vi "HB_ThreadPool.MainDFSMTask.vi"() -> ()   [LabVIEW 2009, in "HGF_DIM_DFSM_Examples.lvlib"]
doc: "Simple application to test the HGF_ThreadPool with a simple class."
uses:
  HGF_DIM_DFSM_Examples.lvlib
  lib.lib/HGF_LVC/HGF_StateCharts/HGF_DeviceFSM/HGF_DeviceFSM_Internals.ctl
  lib.lib/HGF_LVC/HGF_StateCharts/HGF_DeviceFSM/HGF_DeviceFSM.lvsc/StatechartState.ctl
  lib.lib/HGF_LVC/HGF_StateCharts/HGF_DeviceFSM/HGF_DeviceFSM.lvsc/State.ctl
  NInstrSim/Factory/HB_DeviceFactory.lvclass
  lib.lib/HGF_LVC/HGF_BaseClasses/HGF_Factory/HGF_Factory.lvclass
  lib.lib/HGF_LVC/HGF_BaseClasses/HGF_Event/HGF_Event.lvclass
  lib.lib/HGF_LVC/HGF_BaseClasses/HGF_ThreadTask/HGF_ThreadTask.lvclass
  lib.lib/HGF_LVC/HGF_BaseClasses/HGF_NetworkVisitor/HGF_NetworkVisitor.lvclass
  lib.lib/HGF_LVC/HGF_BaseClasses/HGF_PVSubscriber/HGF_PVSubscriber.lvclass
  lib.lib/HGF_LVC/HGF_DeviceBaseClasses/HGF_DeviceVisitor/HGF_DeviceVisitor.lvclass
  lib.lib/HGF_LVC/HGF_DIM/HGF_DIMDataConverter/HGF_DIMDataConverter.lvclass
  lib.lib/HGF_LVC/HGF_DIM/HGF_DIMService/HGF_DIMService.lvclass
  lib.lib/HGF_LVC/HGF_DIM/HGF_DIMFactory/HGF_DIMFactory.lvclass/HGF_DIMFactory.lvclass
  NInstrSim/Visitors/NInstrSim_Visitor.lvclass
  lib.lib/HGF_LVC/HGF_BaseClasses/HGF_TriggeredEvent/HGF_TriggeredEvent.lvclass
  lib.lib/HGF_LVC/HGF_BaseClasses/HGF_VariantDataObject/HGF_VariantDataObject.lvclass
  lib.lib/HGF_LVC/HGF_StateCharts/HGF_DeviceFSM/HGF_DeviceFSM.lvsc/Trigger.ctl
  lib.lib/HGF_LVC/HGF_StateCharts/HGF_DFSMFactory/HGF_DFSMFactory.lvclass
  NInstrSim/Visitors/NInstrSim_ReadStatus/NInstrSim_ReadStatus.lvclass
  lib.lib/HGF_LVC/HGF_BaseClasses/HGF_Exception/HGF_Exception.lvclass
  lib.lib/HGF_LVC/HGF_BaseClasses/HGF_ThreadPool/HGF_ThreadPool.lvclass
  lib.lib/HGF_LVC/HGF_BaseClasses/HGF_Reference/HGF_Reference.lvclass
  lib.lib/HGF_LVC/HGF_Auxiliary/HGF_Auxiliary.lvlib
  lib.lib/HGF_LVC/HGF_BaseClasses/HGF_NetworkEvent/HGF_NetworkEvent.lvclass/HGF_NetworkEvent.lvclass
  lib.lib/HGF_LVC/HGF_DIM/HGF_DIMCommand/HGF_DIMCommand.lvclass
  lib.lib/DimLVEvent/LVDimInterface/LVDimInterface.lvlib
  lib.lib/HGF_LVC/HGF_DeviceBaseClasses/HGF_VISADevice/HGF_VISADevice.lvclass
  lib.lib/HGF_LVC/HGF_DeviceBaseClasses/HGF_DeviceBase/HGF_DeviceBase.lvclass
  NInstrSim/NInstrSim.lvclass
  NInstrSim/Visitors/NInstrSim_ConfigureWaveformType/NInstrSim_ConfigureWaveformType.lvclass
  lib.lib/HGF_LVC/HGF_BaseClasses/HGF_PVBase/HGF_PVBase.lvclass
  lib.lib/HGF_LVC/HGF_DIM/HGF_DIMSubscriber/HGF_DIMSubscriber.lvclass
  lib.lib/HGF_LVC/HGF_BaseClasses/HGF_Visitor/HGF_Visitor.lvclass
  lib.lib/HGF_LVC/HGF_StateCharts/HGF_DeviceFSM/HGF_DeviceFSM.lvsc
  lib.lib/HGF_LVC/HGF_StateCharts/HGF_TaskDFSM/HGF_TaskDFSM.lvclass
  lib.lib/HGF_LVC/HGF_StateCharts/HGF_DFSMVisitor/HGF_DFSMVisitor.lvclass
  lib.lib/HGF_LVC/HGF_DeviceBaseClasses/HGF_DeviceBaseClasses.lvlib
panel:
  out "Active States":T1
  out "internals":T3
  out "error code":i32
  out "no link":bool
  in  "getStatus":bool
  in  "Trigger":T4
  in  "autoConfigure":bool=TRUE
  out "exception":errorcluster
  in  "function (0:Sine)":u16(ring) items=["Sine", "Square", "Sine+Noise", "Random", "Chirp"]
  in  "Serial Configuration":T5={"Baud Rate"=9600, "Flow Control"=0, "Parity"=0, "Data Bits"=7, "Stop Bits"=10} {"Stop Bits" items=["1.0"=10, "1.5"=15, "2.0"=20]; "Data Bits" items=["7"=7, "8"=8]; "Parity" items=["None", "Odd", "Even", "Mark", "Space"]; "Flow Control" items=["None"=0, "XON/XOFF"=1, "RTS/CTS"=2, "DTR/DSR"=4]; "Baud Rate" items=["300"=300, "600"=600, "1200"=1200, "2400"=2400, "4800"=4800, "9600"=9600, "19200"=19200]}
  in  "VISA Resource Name":refnum<visa-resource-name>="GPIB0::13::INSTR"
  in  "objectName":string="myInstrSim"
  out "dcMeasurement":dbl format="%_6g"
  out "Waveform Graph":waveform(dbl)(graph)
  in  "timeout in ms (-1)":i32=3000
  out "nofTasksInQueueOut":i32
  out "nofTasksWaiting":i32
  out "autoIncrementLimit":i32=-1
  out "nofThreads":i32
  out "Default Destination timed out?":bool
  out "got object?":bool
  out "error":errorcluster
  in  "stop":bool
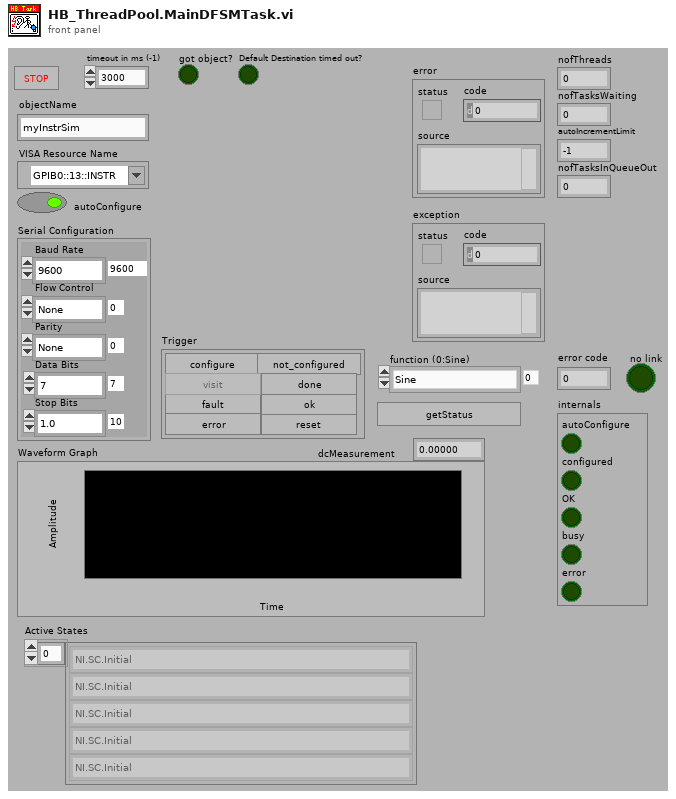
[diagram p1: front panel]
types:
  T1 = typedef "HGF_DeviceFSM.lvlib/HGF_DeviceFSM.lvsc/StatechartState.ctl" = T2[]
  T2 = typedef "HGF_DeviceFSM.lvlib/HGF_DeviceFSM.lvsc/State.ctl" = enum16{"NI.SC.Initial", "NI.SC.History", "NI.SC.ShallowHistory", "NI.SC.Terminal", "Alive", "Alive\\LiveCycle\\Configure", "Alive\\LiveCycle\\Configured", "Alive\\LiveCycle\\Error", "Alive\\LiveCycle\\NotConfigured", "Alive\\LiveCycle\\Configured\\ConfiguredRegion\\Busy", "Alive\\LiveCycle\\Configured\\ConfiguredRegion\\Idle", "Alive\\LiveCycle\\Configured\\ConfiguredRegion\\Idle\\IdleRegion\\Fault", "Alive\\LiveCycle\\Configured\\ConfiguredRegion\\Idle\\IdleRegion\\OK"}
  T3 = typedef "HGF_DeviceBaseClasses.lvlib/HGF_DeviceFSM_Internals.ctl" = cluster{"autoConfigure":bool, "configured":bool, "OK":bool, "busy":bool, "error":bool}
  T4 = cluster{"configure":bool, "visit":bool, "ok":bool, "resetError":bool, "not_configured":bool, "done":bool, "fault":bool, "error":bool}
  T5 = cluster{"Baud Rate":u32, "Flow Control":u16, "Parity":u16, "Data Bits":u16, "Stop Bits":u16}
  T6 = typedef "HGF_DeviceFSM.lvlib/HGF_DeviceFSM.lvsc/Trigger.ctl" = enum16{"NULL", "configure", "fault", "error", "resetError", "STOP", "visit", "not_configured", "done", "ok", "previsit", "configured"}
  T7 = cluster{"Boolean array[0]":bool, "Boolean array[1]":bool, "Boolean array[2]":bool, "Boolean array[3]":bool, "Boolean array[4]":bool}
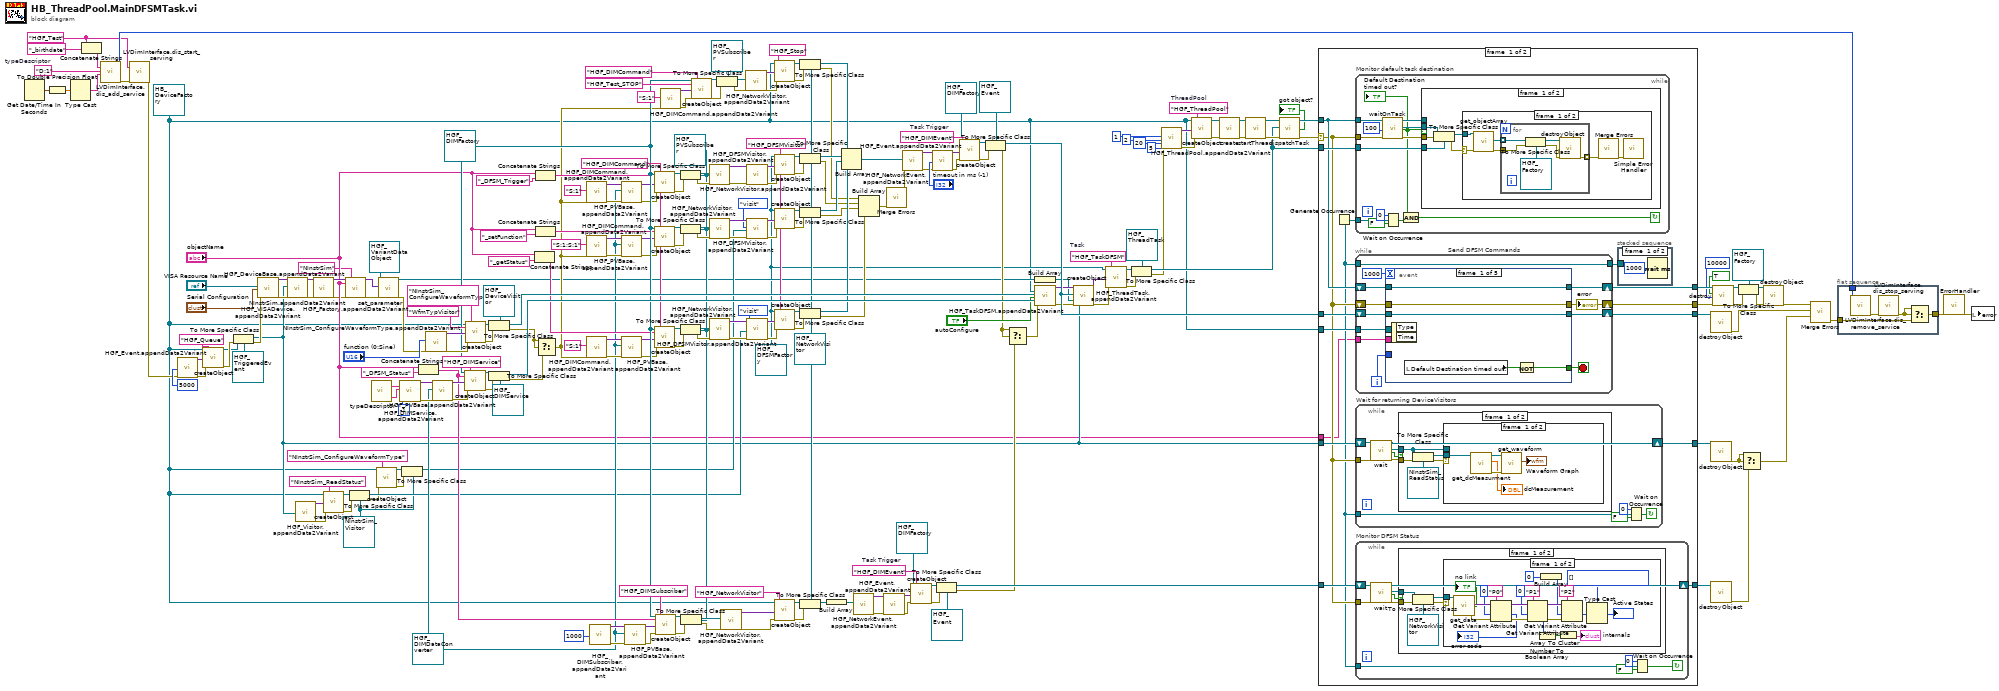
[diagram p0: block diagram]
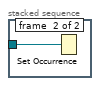
[diagram p4: hidden frame]
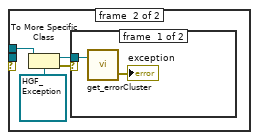
[diagram p5: hidden frame]
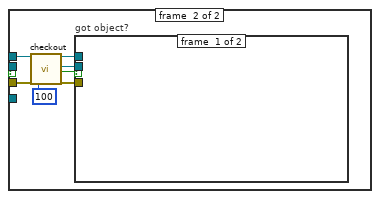
[diagram p9: hidden frame]
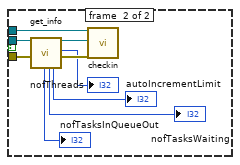
[diagram p10: hidden frame]
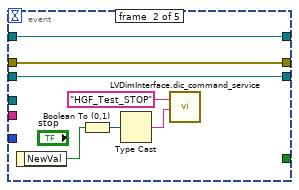
[diagram p11: hidden frame]
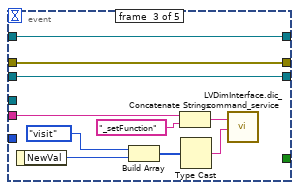
[diagram p12: hidden frame]
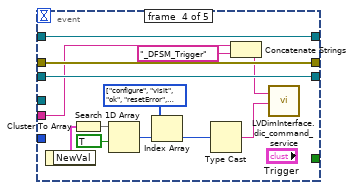
[diagram p13: hidden frame]
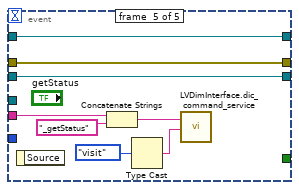
[diagram p14: hidden frame]
diagram:
  w2 = refnum<class "HGF_DFSMFactory.lvclass"> refnum ("HGF_DeviceFSM.lvlib:HGF_DFSMFactory.lvclass")
  w26 = refnum<class "NInstrSim_Visitor.lvclass"> refnum ("HB_HGF_Test.lvlib:NInstrSim_Visitor.lvclass")
  w72 = "HGF_DIMEvent"  # Task Trigger
  w58 = refnum<class "HGF_DIMFactory.lvclass"> refnum ("HGF_DIM.lvlib:HGF_DIMFactory.lvclass")
  w60 = refnum<class "HGF_PVSubscriber.lvclass"> refnum ("HGF_PVSubscriber")
  w103 = "HGF_DIMCommand" ("className")
  w90 = "HGF_DFSMVisitor" ("className")
  w35 = refnum<class "HGF_DIMDataConverter.lvclass"> refnum ("HGF_DIM.lvlib:HGF_DIMBaseType.lvclass")
  w177 = "HGF_Test" ("serverName")
  w182 = "D:1"  # typeDescriptor
  w77 = refnum<class "HGF_NetworkVisitor.lvclass"> refnum ("HGF_BaseClasses.lvlib:HGF_NetworkData.lvclass")
  w230 = "HGF_DIMEvent"  # Task Trigger
  w229 = "HGF_TaskDFSM"  # Task
  w222 = "HGF_ThreadPool"  # ThreadPool
  w1 = refnum<class "HB_DeviceFactory.lvclass"> refnum ("HB_Factory.lvclass")
  n1 = Get Date/Time In Seconds() -> (seconds since 1Jan1904=w180:timestamp)
  n2 = To Double Precision Float(number=w180) -> (double precision float=w181:dbl)
  n3 = Type Cast(x=w181) -> (*(type *) &x=w183:string)  [unwired: 1 out]
  n4 = Concatenate Strings(w177, "_birthdate") -> (w176:string)
  n5 = call "LVDimInterface.dis_add_service.vi"("serviceName"=w176, "typeDescriptor"=w182, "data"=w183) -> ("my_serviceID"=w179:i32, "error out"=w184:errorcluster)  [unwired: 2 in, 13 out]
  n6 = call "LVDimInterface.dis_start_serving.vi"("serverName"=w177, "error in (no error)"=w184) -> ("error out"=w154:errorcluster)  [unwired: 17 out]
  n7 = call "HGF_Event.appendData2Variant.vi"("timeout in ms (-1)"=5000, "error in (no error)"=w154) -> ("dup initData"=w165:variant, "error out"=w166:errorcluster)  [unwired: 1 in, 15 out]
  n8 = call "createObject.vi"("HGF_Factory"=w1, "initializationData"=w165, "error in (no error)"=w166, "className"="HGF_Queue") -> ("HGF_Object"=w162:refnum<class "HGF_Factory.lvclass">, "error out"=w163:errorcluster)  [unwired: 2 in, 12 out]
  n9 = To More Specific Class(target class=refnum<class "HGF_TriggeredEvent.lvclass"> refnum ("Status_Event"), reference=w162, error in=w163) -> (specific class reference=w21:refnum<class "HGF_TriggeredEvent.lvclass">, error out=w161:errorcluster)
  n10 = call "HGF_VISADevice.appendData2Variant.vi"("VISA Resource Name"="VISA Resource Name", "Serial Configuration"="Serial Configuration", "error in (no error)"=w161) -> ("dup initData"=w171:variant, "error out"=w169:errorcluster)  [unwired: 1 in, 14 out]
  n11 = call "NInstrSim.appendData2Variant.vi"("initData"=w171, "statusEvent"=w21, "error in (no error)"=w169) -> ("dup initData"=w170:variant, "error out"=w168:errorcluster)  [unwired: 15 out]
  n12 = call "HGF_Visitor.appendData2Variant.vi"("destination"=w21) -> ("dup initData"=w23:variant, "error out"=w22:errorcluster)  [unwired: 3 in, 14 out]
  n13 = call "HGF_DeviceBase.appendData2Variant.vi"("initData"=w170, "error in (no error)"=w168) -> ("dup initData"=w16:variant, "error out"=w13:errorcluster)  [unwired: 16 out]
  n14 = call "createObject.vi"("HGF_Factory"=w1, "initializationData"=w23, "error in (no error)"=w22, "className"="NInstrSim_ReadStatus") -> ("HGF_Object"=w34:refnum<class "HGF_Factory.lvclass">, "error out"=w33:errorcluster)  [unwired: 2 in, 12 out]
  n15 = call "HGF_Factory.appendData2Variant.vi"("initData"=w16, "objectName"="objectName", "error in (no error)"=w13, "className"="NInstrSim") -> ("dup initData"=w11:variant, "error out"=w10:errorcluster)  [unwired: 14 out]
  n16 = To More Specific Class(target class=w26, reference=w34, error in=w33) -> (specific class reference=w30:refnum<class "NInstrSim_Visitor.lvclass">, error out=w25:errorcluster)
  n17 = call "typeDescriptor.vi"() -> ("defaultData"=w136:string, "typeDescriptor"=w137:string)
  n18 = call "createObject.vi"("HGF_Factory"=w1, "error in (no error)"=w25, "className"="NInstrSim_ConfigureWaveformType") -> ("HGF_Object"=w31:refnum<class "HGF_Factory.lvclass">, "error out"=w32:errorcluster)  [unwired: 3 in, 12 out]
  n19 = call "set_parameter.vi"("HGF_VariantDataObject"=refnum<class "HGF_VariantDataObject.lvclass"> refnum ("HGF_BaseClasses.lvlib:HGF_VariantDataObject.lvclass"), "Parameter"=w11, "error in (no error)"=w10) -> ("dup HGF_VariantDataObject"=w7:refnum<class "HGF_VariantDataObject.lvclass">, "error out"=w8:errorcluster)  [unwired: 1 in, 14 out]
  n20 = call "HGF_DIMService.appendData2Variant.vi"("typeDescriptor"=w137, "defaultData"=w136, "defaultQuality"=-1) -> ("dup initData"=w147:variant, "error out"=w148:errorcluster)  [unwired: 2 in, 13 out]
  n21 = To More Specific Class(target class=w26, reference=w31, error in=w32) -> (specific class reference=w27:refnum<class "NInstrSim_Visitor.lvclass">)  [unwired: 1 out]
  n22 = Concatenate Strings("objectName", "_DFSM_Status" ("string")) -> (w79:string)
  n23 = call "NInstrSim_ConfigureWaveformType.appendData2Variant.vi"("function (0:Sine)"="function (0:Sine)", "error in (no error)"=w8) -> ("dup initData"=w159:variant, "error out"=w150:errorcluster)  [unwired: 1 in, 15 out]
  n24 = call "HGF_PVBase.appendData2Variant.vi"("initData"=w147, "HGF_PVDataConverter"=w35, "error in (no error)"=w148) -> ("dup initData"=w146:variant, "error out"=w145:errorcluster)  [unwired: 15 out]
  n25 = call "createObject.vi"("HGF_Factory"=w58, "objectName"=w79, "initializationData"=w146, "error in (no error)"=w145, "className"="HGF_DIMService") -> ("HGF_Object"=w141:refnum<class "HGF_Factory.lvclass">, "error out"=w140:errorcluster)  [unwired: 1 in, 12 out]
  n26 = call "createObject.vi"("HGF_Factory"=w1, "objectName"="WfmTypVisitor", "initializationData"=w159, "error in (no error)"=w150, "className"="NInstrSim_ConfigureWaveformType") -> ("HGF_Object"=w158:refnum<class "HGF_Factory.lvclass">, "error out"=w160:errorcluster)  [unwired: 13 out]
  n27 = To More Specific Class(target class=refnum<class "HGF_DeviceVisitor.lvclass"> refnum ("HGF_DeviceBaseClasses.lvlib:HGF_DeviceVisitor.lvclass"), reference=w158, error in=w160) -> (specific class reference=w151:refnum<class "HGF_DeviceVisitor.lvclass">, error out=w134:errorcluster)
  n28 = To More Specific Class(target class=refnum<class "HGF_DIMService.lvclass"> refnum ("HGF_DIM.lvlib:HGF_DIMService.lvclass"), reference=w141, error in=w140) -> (specific class reference=w138:refnum<class "HGF_DIMService.lvclass">, error out=w135:errorcluster)
  n29 = Concatenate Strings("objectName", "_getStatus" ("objectName")) -> (w52:string)
  n30 = Concatenate Strings("objectName", "_DFSM_Trigger" ("objectName")) -> (w56:string)
  n31 = Concatenate Strings("objectName", "_setFunction" ("objectName")) -> (w54:string)
  n32 = Select(t=w134, s=w134, f=w135) -> (s? t:f=w50:errorcluster)
  n33 = call "HGF_DIMCommand.appendData2Variant.vi"("typeDescriptor"="S:1", "error in (no error)"=w50) -> ("dup initData"=w37:variant, "error out"=w36:errorcluster)  [unwired: 1 in, 15 out]
  n34 = call "HGF_DIMCommand.appendData2Variant.vi"("typeDescriptor"="S:1;S:1", "error in (no error)"=w50) -> ("dup initData"=w43:variant, "error out"=w42:errorcluster)  [unwired: 1 in, 15 out]
  n35 = call "HGF_DIMCommand.appendData2Variant.vi"("typeDescriptor"="S:1", "error in (no error)"=w50) -> ("dup initData"=w47:variant, "error out"=w45:errorcluster)  [unwired: 1 in, 15 out]
  n36 = call "HGF_DIMSubscriber.appendData2Variant.vi"("timeout [0s]"=1000) -> ("dup initData"=w88:variant, "error out"=w89:errorcluster)  [unwired: 4 in, 13 out]
  n37 = call "HGF_PVBase.appendData2Variant.vi"("initData"=w37, "HGF_PVDataConverter"=w35, "error in (no error)"=w36) -> ("dup initData"=w39:variant, "error out"=w38:errorcluster)  [unwired: 15 out]
  n38 = call "HGF_PVBase.appendData2Variant.vi"("initData"=w43, "HGF_PVDataConverter"=w35, "error in (no error)"=w42) -> ("dup initData"=w41:variant, "error out"=w40:errorcluster)  [unwired: 15 out]
  n39 = call "HGF_PVBase.appendData2Variant.vi"("initData"=w47, "HGF_PVDataConverter"=w35, "error in (no error)"=w45) -> ("dup initData"=w46:variant, "error out"=w44:errorcluster)  [unwired: 15 out]
  n40 = call "HGF_PVBase.appendData2Variant.vi"("initData"=w88, "HGF_PVDataConverter"=w35, "error in (no error)"=w89) -> ("dup initData"=w86:variant, "error out"=w87:errorcluster)  [unwired: 15 out]
  n41 = call "createObject.vi"("HGF_Factory"=w58, "objectName"=w56, "initializationData"=w39, "error in (no error)"=w38, "className"=w103) -> ("HGF_Object"=w133:refnum<class "HGF_Factory.lvclass">, "error out"=w99:errorcluster)  [unwired: 1 in, 12 out]
  n42 = call "createObject.vi"("HGF_Factory"=w58, "objectName"=w54, "initializationData"=w41, "error in (no error)"=w40, "className"=w103) -> ("HGF_Object"=w115:refnum<class "HGF_Factory.lvclass">, "error out"=w98:errorcluster)  [unwired: 1 in, 12 out]
  n43 = call "createObject.vi"("HGF_Factory"=w58, "objectName"=w52, "initializationData"=w46, "error in (no error)"=w44, "className"=w103) -> ("HGF_Object"=w114:refnum<class "HGF_Factory.lvclass">, "error out"=w97:errorcluster)  [unwired: 1 in, 12 out]
  n44 = call "createObject.vi"("HGF_Factory"=w58, "objectName"=w79, "initializationData"=w86, "error in (no error)"=w87, "className"="HGF_DIMSubscriber") -> ("HGF_Object"=w81:refnum<class "HGF_Factory.lvclass">, "error out"=w82:errorcluster)  [unwired: 1 in, 12 out]
  n45 = call "HGF_DIMCommand.appendData2Variant.vi"("typeDescriptor"="S:1", "error in (no error)"=w50) -> ("dup initData"=w198:variant, "error out"=w100:errorcluster)  [unwired: 1 in, 15 out]
  n46 = To More Specific Class(target class=w60, reference=w133, error in=w99) -> (specific class reference=w129:refnum<class "HGF_PVSubscriber.lvclass">, error out=w132:errorcluster)
  n47 = To More Specific Class(target class=w60, reference=w115, error in=w98) -> (specific class reference=w117:refnum<class "HGF_PVSubscriber.lvclass">, error out=w116:errorcluster)
  n48 = To More Specific Class(target class=w60, reference=w114, error in=w97) -> (specific class reference=w112:refnum<class "HGF_PVSubscriber.lvclass">, error out=w113:errorcluster)
  n49 = To More Specific Class(target class=w60, reference=w81, error in=w82) -> (specific class reference=w85:refnum<class "HGF_PVSubscriber.lvclass">, error out=w61:errorcluster)
  n50 = call "createObject.vi"("HGF_Factory"=w58, "objectName"="HGF_Test_STOP", "initializationData"=w198, "error in (no error)"=w100, "className"="HGF_DIMCommand") -> ("HGF_Object"=w194:refnum<class "HGF_Factory.lvclass">, "error out"=w195:errorcluster)  [unwired: 1 in, 12 out]
  n51 = call "HGF_NetworkVisitor.appendData2Variant.vi"("HGF_PVSubscriber"=w129, "error in (no error)"=w132) -> ("dup initData"=w126:variant, "error out"=w124:errorcluster)  [unwired: 1 in, 15 out]
  n52 = call "HGF_NetworkVisitor.appendData2Variant.vi"("HGF_PVSubscriber"=w117, "error in (no error)"=w116) -> ("dup initData"=w119:variant, "error out"=w121:errorcluster)  [unwired: 1 in, 15 out]
  n53 = call "HGF_NetworkVisitor.appendData2Variant.vi"("HGF_PVSubscriber"=w112, "error in (no error)"=w113) -> ("dup initData"=w111:variant, "error out"=w109:errorcluster)  [unwired: 1 in, 15 out]
  n54 = To More Specific Class(target class=refnum<class "HGF_PVSubscriber.lvclass"> refnum ("HGF_PVSubscriber"), reference=w194, error in=w195) -> (specific class reference=w202:refnum<class "HGF_PVSubscriber.lvclass">, error out=w196:errorcluster)
  n55 = call "HGF_NetworkVisitor.appendData2Variant.vi"("HGF_PVSubscriber"=w85, "error in (no error)"=w61) -> ("dup initData"=w49:variant, "error out"=w48:errorcluster)  [unwired: 1 in, 15 out]
  n56 = call "HGF_NetworkVisitor.appendData2Variant.vi"("HGF_PVSubscriber"=w202, "error in (no error)"=w196) -> ("dup initData"=w190:variant, "error out"=w189:errorcluster)  [unwired: 1 in, 15 out]
  n57 = call "HGF_DFSMVisitor.appendData2Variant.vi"("initData"=w126, "error in (no error)"=w124) -> ("dup initData"=w125:variant, "error out"=w123:errorcluster)  [unwired: 2 in, 14 out]
  n58 = call "HGF_DFSMVisitor.appendData2Variant.vi"("initData"=w119, "trigger"=Trigger."visit", "deviceVisitor"=w27, "error in (no error)"=w121) -> ("dup initData"=w120:variant, "error out"=w122:errorcluster)  [unwired: 14 out]
  n59 = call "HGF_DFSMVisitor.appendData2Variant.vi"("initData"=w111, "trigger"=Trigger."visit", "deviceVisitor"=w30, "error in (no error)"=w109) -> ("dup initData"=w110:variant, "error out"=w108:errorcluster)  [unwired: 14 out]
  n60 = call "createObject.vi"("HGF_Factory"=w1, "initializationData"=w190, "error in (no error)"=w189, "className"="HGF_Stop") -> ("HGF_Object"=w200:refnum<class "HGF_Factory.lvclass">, "error out"=w201:errorcluster)  [unwired: 2 in, 12 out]
  n61 = call "createObject.vi"("HGF_Factory"=w2, "initializationData"=w125, "error in (no error)"=w123, "className"=w90) -> ("HGF_Object"=w131:refnum<class "HGF_Factory.lvclass">, "error out"=w130:errorcluster)  [unwired: 2 in, 12 out]
  n62 = call "createObject.vi"("HGF_Factory"=w2, "initializationData"=w120, "error in (no error)"=w122, "className"=w90) -> ("HGF_Object"=w107:refnum<class "HGF_Factory.lvclass">, "error out"=w106:errorcluster)  [unwired: 2 in, 12 out]
  n63 = call "createObject.vi"("HGF_Factory"=w2, "initializationData"=w110, "error in (no error)"=w108, "className"=w90) -> ("HGF_Object"=w105:refnum<class "HGF_Factory.lvclass">, "error out"=w104:errorcluster)  [unwired: 2 in, 12 out]
  n64 = call "createObject.vi"("HGF_Factory"=w1, "initializationData"=w49, "error in (no error)"=w48, "className"="HGF_NetworkVisitor") -> ("HGF_Object"=w84:refnum<class "HGF_Factory.lvclass">, "error out"=w83:errorcluster)  [unwired: 2 in, 12 out]
  n65 = To More Specific Class(target class=w77, reference=w200, error in=w201) -> (specific class reference=w191:refnum<class "HGF_NetworkVisitor.lvclass">, error out=w94:errorcluster)
  n66 = To More Specific Class(target class=w77, reference=w131, error in=w130) -> (specific class reference=w128:refnum<class "HGF_NetworkVisitor.lvclass">, error out=w93:errorcluster)
  n67 = To More Specific Class(target class=w77, reference=w107, error in=w106) -> (specific class reference=w102:refnum<class "HGF_NetworkVisitor.lvclass">, error out=w92:errorcluster)
  n68 = To More Specific Class(target class=w77, reference=w105, error in=w104) -> (specific class reference=w101:refnum<class "HGF_NetworkVisitor.lvclass">, error out=w91:errorcluster)
  n69 = To More Specific Class(target class=w77, reference=w84, error in=w83) -> (specific class reference=w68:refnum<class "HGF_NetworkVisitor.lvclass">)  [unwired: 1 out]
  n70 = Build Array(w68) -> (w67:refnum<class "HGF_NetworkVisitor.lvclass">[])
  n71 = Build Array(w191, w128, w102, w101) -> (w203:refnum<class "HGF_NetworkVisitor.lvclass">[])
  n72 = call "HGF_NetworkEvent.appendData2Variant.vi"("callbackVisitors"=w67) -> ("dup initData"=w75:variant, "error out"=w76:errorcluster)  [unwired: 2 in, 15 out]
  n73 = Build Array(w94, w93, w92, w91) -> (w95:errorcluster[])
  n74 = call "HGF_Event.appendData2Variant.vi"("initData"=w75, "error in (no error)"=w76) -> ("dup initData"=w70:variant, "error out"=w71:errorcluster)  [unwired: 2 in, 14 out]
  n75 = call <vilib>:"Merge Errors.vi"("error array in"=w95) -> ("error out"=w96:errorcluster)  [unwired: 3 in, 3 out]
  n76 = call "HGF_NetworkEvent.appendData2Variant.vi"("callbackVisitors"=w203, "error in (no error)"=w96) -> ("dup initData"=w205:variant, "error out"=w204:errorcluster)  [unwired: 1 in, 15 out]
  n77 = call "createObject.vi"("HGF_Factory"=refnum<class "HGF_DIMFactory.lvclass"> refnum ("HGF_DIM.lvlib:HGF_DIMFactory.lvclass"), "initializationData"=w70, "error in (no error)"=w71, "className"=w72) -> ("HGF_Object"=w73:refnum<class "HGF_Factory.lvclass">, "error out"=w69:errorcluster)  [unwired: 2 in, 12 out]
  n78 = call "HGF_Event.appendData2Variant.vi"("initData"=w205, "timeout in ms (-1)"="timeout in ms (-1)", "error in (no error)"=w204) -> ("dup initData"=w235:variant, "error out"=w234:errorcluster)  [unwired: 1 in, 14 out]
  n79 = To More Specific Class(target class=refnum<class "HGF_Event.lvclass"> refnum ("HGF_BaseClasses.lvlib:HGF_Event.lvclass"), reference=w73, error in=w69) -> (specific class reference=w66:refnum<class "HGF_Event.lvclass">, error out=w64:errorcluster)
  n80 = call "createObject.vi"("HGF_Factory"=refnum<class "HGF_DIMFactory.lvclass"> refnum ("HGF_DIM.lvlib:HGF_DIMFactory.lvclass"), "initializationData"=w235, "error in (no error)"=w234, "className"=w230) -> ("HGF_Object"=w227:refnum<class "HGF_Factory.lvclass">, "error out"=w236:errorcluster)  [unwired: 2 in, 12 out]
  n81 = To More Specific Class(target class=refnum<class "HGF_Event.lvclass"> refnum ("HGF_BaseClasses.lvlib:HGF_Event.lvclass"), reference=w227, error in=w236) -> (specific class reference=w212:refnum<class "HGF_Event.lvclass">, error out=w63:errorcluster)
  n82 = Select(t=w63, s=w63, f=w64) -> (s? t:f=w62:errorcluster)
  n83 = Build Array(w7) -> (w12:refnum<class "HGF_VariantDataObject.lvclass">[])
  n84 = call "HGF_TaskDFSM.appendData2Variant.vi"("deviceFactory"=w1, "autoConfigVisitor"=w151, "autoConfigure"="autoConfigure", "statusPublisher"=w138, "error in (no error)"=w62) -> ("dup initData"=w152:variant, "error out"=w153:errorcluster)  [unwired: 1 in, 12 out]
  n85 = call "HGF_ThreadTask.appendData2Variant.vi"("initData"=w152, "taskTrigger"=w212, "objectArray"=w12, "error in (no error)"=w153, "exceptionEvent"=w21) -> ("dup initData"=w221:variant, "error out"=w220:errorcluster)  [unwired: 1 in, 12 out]
  n86 = call "createObject.vi"("HGF_Factory"=w2, "initializationData"=w221, "error in (no error)"=w220, "className"=w229) -> ("HGF_Object"=w226:refnum<class "HGF_Factory.lvclass">, "error out"=w233:errorcluster)  [unwired: 2 in, 12 out]
  n87 = To More Specific Class(target class=refnum<class "HGF_ThreadTask.lvclass"> refnum ("HGF_BaseClasses.lvlib:HGF_ThreadTask.lvclass"), reference=w226, error in=w233) -> (specific class reference=w213:refnum<class "HGF_ThreadTask.lvclass">, error out=w208:errorcluster)
  n88 = call "HGF_ThreadPool.appendData2Variant.vi"("initialNofThreads (0)"=1 ("initialNofThreads"), "incThreads(1)"=2 ("incThreads"), "maxNofThreads (-1:unlimited)"=20 ("maxNofThreads"), "error in (no error)"=w208, "autoIncrementLimit (-1)"=5) -> ("dup initData"=w247:variant, "error out"=w209:errorcluster)  [unwired: 2 in, 11 out]
  n89 = call "createObject.vi"("HGF_Factory"=w1, "initializationData"=w247, "error in (no error)"=w209, "className"=w222) -> ("HGF_Object"=w228:refnum<class "HGF_Factory.lvclass">, "error out"=w246:errorcluster)  [unwired: 2 in, 12 out]
  n90 = call "create.vi"("Object"=w228, "error in (no error)"=w246) -> ("HGF_Reference"=w248:refnum<class "HGF_Reference.lvclass">, "error out"=w242:errorcluster)  [unwired: 1 in, 15 out]
  n91 = call "startThread.vi"("HGF_ThreadPool_Reference"=w248, "error in (no error)"=w242) -> ("dup HGF_ThreadPool_Reference"=w218:refnum<class "HGF_Reference.lvclass">, "error out"=w216:errorcluster)  [unwired: 1 in, 15 out]
  n92 = call "dispatchTask.vi"("HGF_ThreadPool_Reference"=w218, "HGF_ThreadTask"=w213, "error in (no error)"=w216) -> ("dup HGF_ThreadPool_Reference"=w217:refnum<class "HGF_Reference.lvclass">, "got object?"=→"got object?":bool, "error out"=w215:errorcluster)  [unwired: 1 in, 13 out]
  n93 = case shown="No Error" w215 {
    selector: w215 -> [w252 w433]
    tunnel: w217 -> [w260 w434]
    tunnel: [w263 w434] -> w232
    tunnel: w213 -> [w261 _]
    tunnel: [w262 w433] -> w231
    tunnel: w212 -> [w256 w431]
    tunnel: w21 -> [w257 w432]
    tunnel: w1 -> [w258 _]
    tunnel: [w255 w432] -> w207
    tunnel: [w254 w431] -> w206
    tunnel: w66 -> [w253 w430]
    tunnel: "objectName" -> [w250 _]
    tunnel: [w249 w430] -> w20
    frame #0 {
      n94 = Generate Occurrence() -> (w251:refnum<k4>)
      n95 = while "Monitor default task destination" {
        tunnel: w261 -> [w338]
        tunnel: w260 -> [w337]
        tunnel: w252 -> [w336]
        tunnel: w251 -> [w332]
        stop <- w329 continue-if-true
        n96 = call "waitOnTask.vi"("HGF_ThreadPool_Reference"=w337, "timeout in ms (-1)"=100, "error in (no error)"=w336) -> ("dup HGF_ThreadPool_Reference"=w341:refnum<class "HGF_Reference.lvclass">, "HGF_Task"=w340:refnum<class "HGF_ThreadTask.lvclass">, "timed out?"=w331:bool, "error out"=w335:errorcluster)  [unwired: 13 out]
        "Default Destination timed out?" <- w331
        n97 = Wait on Occurrence(1:FALSE ("ignore previous (T)"), 2:w332, 3:0 ("ms timeout (-1)")) -> (0:w330:bool)
        n98 = And(x=w331, y=w330) -> (x .and. y?=w329:bool)
        n99 = case "timed out?" shown="False" w331 {
          tunnel: w340 -> [w346 _]
          tunnel: w335 -> [w345 w359]
          tunnel: w341 -> [_ w360]
          tunnel: w338 -> [w342 _]
          frame #0 {
            n100 = To More Specific Class(target class=w342, reference=w346, error in=w345) -> (specific class reference=w344:refnum<class "HGF_ThreadTask.lvclass">, error out=w343:errorcluster)
            n101 = case shown="No Error" w343 {
              selector: w343 -> [w351 _]
              tunnel: w344 -> [w352 _]
              frame #0 {
                n102 = call "get_objectArray.vi"("HGF_ThreadTask"=w352, "error in (no error)"=w351) -> ("objectArray"=w347:refnum<class>[], "error out"=w349:errorcluster)  [unwired: 16 out]
                n103 = for {
                  tunnel: w349 -> [w354]
                  tunnel: [w358] -> w350 mode=indexing
                  tunnel: w347 -> [w355] mode=indexing
                  n104 = To More Specific Class(target class=refnum<class "HGF_Factory.lvclass"> refnum ("HGF_BaseClasses.lvlib:HGF_Factory.lvclass"), reference=w355, error in=w354) -> (specific class reference=w353:refnum<class "HGF_Factory.lvclass">, error out=w356:errorcluster)
                  n105 = call "destroyObject.vi"("HGF_Factory"=w353, "error in (no error)"=w356) -> ("error out"=w358:errorcluster)  [unwired: 17 out]
                }
                n106 = call <vilib>:"Merge Errors.vi"("error array in"=w350) -> ("error out"=w348:errorcluster)  [unwired: 3 in, 3 out]
                n107 = call <vilib>:"Simple Error Handler.vi"("error in (no error)"=w348) -> ()  [unwired: 1 in, 8 out]
              }
              frame #1 {
              }
            }
          }
          frame #1 {
            n108 = call "checkout.vi"("HGF_ThreadPool_Reference"=w360, "timeout in ms (-1)"=100, "error in (no error)"=w359) -> ("dup HGF_ThreadPool_Reference"=w361:refnum<class "HGF_Reference.lvclass">, "HGF_ThreadPool"=w362:refnum<class "HGF_ThreadPool.lvclass">, "got object?"=w365:bool, "error out"=w363:errorcluster)  [unwired: 13 out]
            n109 = case "got object?" shown="True" w365 {
              tunnel: w361 -> [_ w374]
              tunnel: w362 -> [_ w373]
              tunnel: w363 -> [_ w372]
              frame #0 {
              }
              frame #1 {
                n110 = call "get_info.vi"("HGF_ThreadPool"=w373, "error in (no error)"=w372) -> ("nofTasksInQueueOut"=→"nofTasksInQueueOut":i32, "nofTasksWaiting"=→"nofTasksWaiting":i32, "autoIncrementLimit"=→"autoIncrementLimit":i32, "dup HGF_ThreadPool"=w370:refnum<class "HGF_ThreadPool.lvclass">, "nofThreads"=→"nofThreads":i32, "error out"=w371:errorcluster)  [unwired: 12 out]
                n111 = call "checkin.vi"("HGF_Reference"=w374, "Object"=w370, "error in (no error)"=w371) -> ()  [unwired: 1 in, 16 out]
              }
            }
          }
        }
      }
      n112 = while "Send DFSM Commands" {
        shift-right: [w385] -> w263
        shift-left: w260 -> [w384]
        shift-right: [w377] -> w262
        shift-left: w252 -> [w386]
        tunnel: w251 -> [w381]
        tunnel: [w381] -> w259
        tunnel: w258 -> [w382]
        shift-right: [w379] -> w254
        shift-left: w256 -> [w383]
        tunnel: w250 -> [w376]
        i -> [w378]
        stop <- w380 stop-if-true
        n113 = event shown="[3] \"Trigger\": Value Change" {
          selector: _ -> [_ _ _ _ _]
          dyn-events: _ -> [_ _ _ _ _]
          timeout: 1000 -> [_ _ _ _ _]
          tunnel: [w387 _ _ _ _] -> w380
          tunnel: [w390 w396 w407 w420 w428] -> w377
          tunnel: w386 -> [w390 w396 w407 w420 w428]
          tunnel: [w391 w398 w408 w421 w429] -> w385
          tunnel: w384 -> [w391 w398 w408 w421 w429]
          tunnel: w383 -> [w389 w397 w406 w419 w427]
          tunnel: w382 -> [_ _ _ _ _]
          tunnel: [w389 w397 w406 w419 w427] -> w379
          tunnel: w378 -> [_ _ _ _ _]
          tunnel: w376 -> [_ _ w403 w411 w425]
          event #0 {
            n114 = event-data() -> ()  [unwired: 3 out]
            n115 = local read "Default Destination timed out?"() -> (w388:bool)
            n116 = Not(x=w388) -> (.not. x?=w387:bool)
          }
          event #1 {
            n117 = event-data() -> ("NewVal"=w394:bool)  [unwired: 1 out]
            n118 = Boolean To (0,1)(Boolean=w394) -> (0, 1=w392:i16)
            n119 = Type Cast(x=w392) -> (*(type *) &x=w393:string)  [unwired: 1 out]
            n120 = call "LVDimInterface.dic_command_service.vi"("commandName"="HGF_Test_STOP" ("objectName"), "data"=w393) -> ()  [unwired: 1 in, 17 out]
          }
          event #2 {
            n121 = event-data() -> ("NewVal"=w401:u16)  [unwired: 1 out]
            n122 = Build Array(Trigger."visit" ("trigger"), w401) -> (w400:u16[])
            n123 = Concatenate Strings(w403, "_setFunction" ("objectName")) -> (w404:string)
            n124 = Type Cast(x=w400) -> (*(type *) &x=w405:string)  [unwired: 1 out]
            n125 = call "LVDimInterface.dic_command_service.vi"("commandName"=w404, "data"=w405) -> ()  [unwired: 1 in, 17 out]
          }
          event #3 {
            w413 = T6[] [enum."configure", enum."visit", enum."ok", enum."resetError", enum."not_configured", enum."done", enum."fault", enum."error"] items=["NULL", "configure", "fault", "error", "resetError", "STOP", "visit", "not_configured", "done", "ok", "previsit", "configured"]
            n126 = event-data() -> ("NewVal"=w414:T4)  [unwired: 1 out]
            n127 = Cluster To Array(cluster=w414) -> (array=w417:bool[])
            n128 = Search 1D Array(1D array=w417, element=TRUE) -> (index of element=w415:i32)  [unwired: 1 out]
            n129 = Index Array(array=w413, index=w415) -> (element=w412:T6)
            n130 = Type Cast(x=w412) -> (*(type *) &x=w418:string)  [unwired: 1 out]
            n131 = Concatenate Strings(w411, "_DFSM_Trigger" ("objectName")) -> (w410:string)
            n132 = call "LVDimInterface.dic_command_service.vi"("commandName"=w410, "data"=w418) -> ()  [unwired: 1 in, 17 out]
          }
          event #4 {
            n133 = event-data() -> ()  [unwired: 2 out]
            n134 = Concatenate Strings(w425, "_getStatus" ("objectName")) -> (w426:string)
            n135 = Type Cast(x=Trigger."visit" ("trigger")) -> (*(type *) &x=w423:string)  [unwired: 1 out]
            n136 = call "LVDimInterface.dic_command_service.vi"("commandName"=w426, "data"=w423) -> ()  [unwired: 1 in, 17 out]
          }
        }
        "error" <- w377
      }
      n137 = while "Wait for returning DeviceVisitors" {
        tunnel: w252 -> [w306]
        tunnel: w251 -> [w309]
        shift-right: [w307] -> w255
        shift-left: w257 -> [w308]
        stop <- w310 continue-if-true
        n138 = call-dynamic "wait.vi"("HGF_Event"=w308, "error in (no error)"=w306) -> ("dup HGF_Event"=w307:refnum<class "HGF_TriggeredEvent.lvclass">, "Object"=w303:refnum<class>, "timed out"=w304:bool, "error out"=w305:errorcluster)  [unwired: 2 in, 12 out]
        n139 = case shown="False" w304 {
          tunnel: w305 -> [w317 _]
          tunnel: w303 -> [w313 _]
          frame #0 {
            n140 = To More Specific Class(target class=refnum<class "NInstrSim_ReadStatus.lvclass"> refnum ("HB_HGF_Test.lvlib:NInstrSim_ReadStatus.lvclass"), reference=w313, error in=w317) -> (specific class reference=w315:refnum<class "NInstrSim_ReadStatus.lvclass">, error out=w316:errorcluster)
            n141 = case shown="No Error" w316 {
              tunnel: w315 -> [w318 _]
              tunnel: w313 -> [_ w323]
              frame #0 {
                n142 = call "get_dcMeasurment.vi"("NInstrSim_ReadStatus"=w318) -> ("dup NInstrSim_ReadStatus"=w320:refnum<class "NInstrSim_ReadStatus.lvclass">, "dcMeasurement"=→"dcMeasurement":dbl, "error out"=w321:errorcluster)  [unwired: 1 in, 15 out]
                n143 = call "get_waveform.vi"("NInstrSim_ReadStatus"=w320, "error in (no error)"=w321) -> ("Waveform"=→"Waveform Graph":waveform(dbl))  [unwired: 17 out]
              }
              frame #1 {
                n144 = To More Specific Class(target class=refnum<class "HGF_Exception.lvclass"> refnum ("HGF_BaseClasses.lvlib:HGF_Exception.lvclass"), reference=w323) -> (specific class reference=w325:refnum<class "HGF_Exception.lvclass">, error out=w324:errorcluster)  [unwired: 1 in]
                n145 = case shown="No Error" w324 {
                  tunnel: w325 -> [w328 _]
                  frame #0 {
                    n146 = call "get_errorCluster.vi"("HGF_Exception"=w328) -> ("errorCluster"=→"exception":errorcluster)  [unwired: 1 out]
                  }
                  frame #1 {
                  }
                }
              }
            }
          }
          frame #1 {
          }
        }
        n147 = Wait on Occurrence(1:FALSE ("ignore previous (T)"), 2:w309, 3:0 ("ms timeout (-1)")) -> (0:w310:bool)
      }
      n148 = while "Monitor DFSM Status" {
        tunnel: w252 -> [w267]
        tunnel: w251 -> [w270]
        shift-right: [w268] -> w249
        shift-left: w253 -> [w269]
        stop <- w271 continue-if-true
        n149 = call-dynamic "wait.vi"("HGF_Event"=w269, "error in (no error)"=w267) -> ("dup HGF_Event"=w268:refnum<class "HGF_Event.lvclass">, "Object"=w264:refnum<class>, "timed out"=w265:bool, "error out"=w266:errorcluster)  [unwired: 2 in, 12 out]
        n150 = case shown="False" w265 {
          tunnel: w266 -> [w278 _]
          tunnel: w264 -> [w277 _]
          frame #0 {
            n151 = To More Specific Class(target class=refnum<class "HGF_NetworkVisitor.lvclass"> refnum ("HGF_BaseClasses.lvlib:HGF_NetworkData.lvclass"), reference=w277, error in=w278) -> (specific class reference=w275:refnum<class "HGF_NetworkVisitor.lvclass">, error out=w276:errorcluster)
            n152 = case shown="No Error" w276 {
              tunnel: w275 -> [w300 _]
              frame #0 {
                w279 = T1 [] items=["NI.SC.Initial", "NI.SC.History", "NI.SC.ShallowHistory", "NI.SC.Terminal", "Alive", "Alive\\LiveCycle\\Configure", "Alive\\LiveCycle\\Configured", "Alive\\LiveCycle\\Error", "Alive\\LiveCycle\\NotConfigured", "Alive\\LiveCycle\\Configured\\ConfiguredRegion\\Busy", "Alive\\LiveCycle\\Configured\\ConfiguredRegion\\Idle", "Alive\\LiveCycle\\Configured\\ConfiguredRegion\\Idle\\IdleRegion\\Fault", "Alive\\LiveCycle\\Configured\\ConfiguredRegion\\Idle\\IdleRegion\\OK"] ("Active States")
                n153 = call "get_data.vi"("HGF_NetworkData"=w300) -> ("data"=w299:variant, "no link"=→"no link":bool, "error out"=w296:errorcluster)  [unwired: 1 in, 15 out]
                n154 = Get Variant Attribute(Variant=w299, name="P0", default value (empty Variant)=0 ("code"), error in=w296) -> (duplicate Variant=w292:variant, value=→"error code":i32, error out=w293:errorcluster)  [unwired: 1 out]
                n155 = Get Variant Attribute(Variant=w292, name="P1", default value (empty Variant)=u32 0 ("code"), error in=w293) -> (duplicate Variant=w289:variant, value=w284:u32, error out=w290:errorcluster)  [unwired: 1 out]
                n156 = Number To Boolean Array(number=w284) -> (Boolean array=w283:bool[])
                n157 = Build Array(u16 0 ("code")) -> (w286:u16[])
                n158 = Array To Cluster(array=w283) -> (cluster=→"internals":T7)
                n159 = Get Variant Attribute(Variant=w289, name="P2", default value (empty Variant)=w286, error in=w290) -> (value=w281:u16[])  [unwired: 3 out]
                n160 = Type Cast(type=w279, x=w281) -> (*(type *) &x=→"Active States":T1)
              }
              frame #1 {
              }
            }
          }
          frame #1 {
          }
        }
        n161 = Wait on Occurrence(1:FALSE ("ignore previous (T)"), 2:w270, 3:0 ("ms timeout (-1)")) -> (0:w271:bool)
      }
      n162 = stacked-sequence {
        tunnel: w259 -> [_ w302]
        frame #0 {
          n163 = Wait (ms)(milliseconds to wait=u32 1000) -> ()  [unwired: 1 out]
        }
        frame #1 {
          n164 = Set Occurrence(w302) -> ()
        }
      }
    }
    frame #1 {
    }
  }
  n165 = call "destroyObject.vi"("HGF_Factory"=w206) -> ("error out"=w187:errorcluster)  [unwired: 1 in, 17 out]
  n166 = call "destroyObject.vi"("HGF_Factory"=w207) -> ("error out"=w18:errorcluster)  [unwired: 1 in, 17 out]
  n167 = call "destroyObject.vi"("HGF_Factory"=w20) -> ("error out"=w19:errorcluster)  [unwired: 1 in, 17 out]
  n168 = call "destroy.vi"("HGF_Reference"=w232, "wait for activity? (F)"=TRUE, "timeout /ms (-1)"=10000, "error in (no error)"=w231) -> ("Object"=w241:refnum<class>, "error out"=w239:errorcluster)  [unwired: 14 out]
  n169 = To More Specific Class(target class=refnum<class "HGF_Factory.lvclass"> refnum ("HGF_BaseClasses.lvlib:HGF_Factory.lvclass"), reference=w241, error in=w239) -> (specific class reference=w240:refnum<class "HGF_Factory.lvclass">, error out=w238:errorcluster)
  n170 = Select(t=w18, s=w18, f=w19) -> (s? t:f=w17:errorcluster)
  n171 = call "destroyObject.vi"("HGF_Factory"=w240, "error in (no error)"=w238) -> ("error out"=w188:errorcluster)  [unwired: 17 out]
  n172 = call <vilib>:"Merge Errors.vi"("error in 3 (no error)"=w17, "error in 2 (no error)"=w187, "error in 1 (no error)"=w188) -> ("error out"=w186:errorcluster)  [unwired: 1 in, 3 out]
  n173 = flat-sequence {
    tunnel: w186 -> [w438]
    tunnel: [w437] -> w185
    tunnel: w179 -> [w435]
    frame #0 {
      n174 = call "LVDimInterface.dis_remove_service.vi"("my_serviceID"=w435) -> ("error out"=w436:errorcluster)  [unwired: 2 in, 16 out]
      n175 = call "LVDimInterface.dis_stop_serving.vi"("error in (no error)"=w436) -> ("error out"=w439:errorcluster)  [unwired: 18 out]
      n176 = Select(t=w439, s=w439, f=w438) -> (s? t:f=w437:errorcluster)
    }
  }
  n177 = call "ErrorHandler.vi"("error in (no error)"=w185) -> ("error out"=w175:errorcluster)  [unwired: 6 in, 12 out]
  n178 = local write "error"(w175) -> ()
